vi "Main.vi"() -> ()   [LabVIEW 2019]
doc: "The myRIO Project template acquires acceleration data from the onboard accelerometer and displays the changes of acceleration values in a waveform chart."
uses:
  D:/PLIKI/INZYNIERKA/PROGRAM/STARE/EnumMS.ctl
panel:
  in  "ROZPOCZNIJ":bool caption="START"
  out "Error":bool
  in  "START":bool
  out "PRZEBIEG PREDKOŚCI OBROTOWEJ":dbl(graph)
  in  "Metody pomiarowe":T1(tab)
  in  "Rozdzielczość":dbl
  in  "Stała napieciowa":dbl
  out "Ścieżka zapisu danych":string
  out "Run":bool
  in  "ZATRZYMAJ":bool
  in  "STOP":bool
  out "Aktualna pedkosć obrotowa":dbl
  in  "Czas pomiaru":dbl
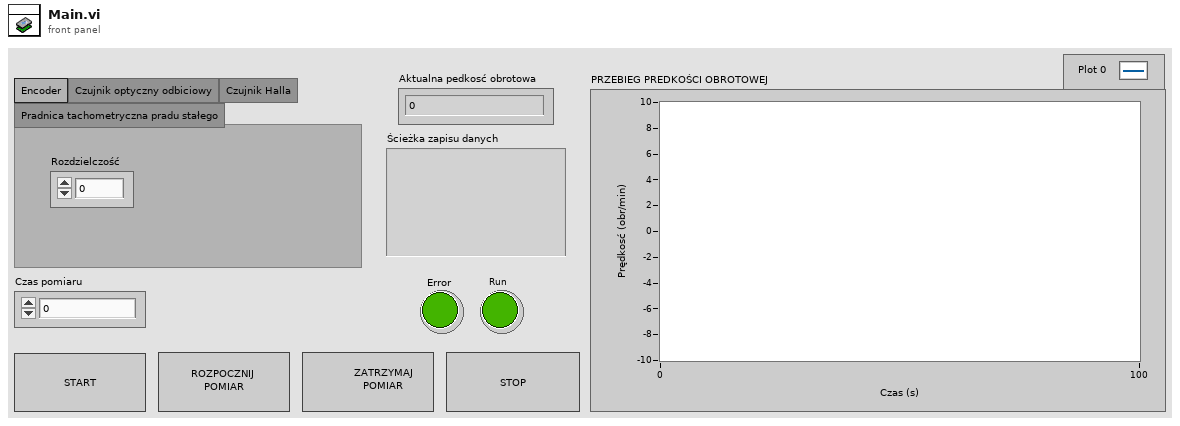
[diagram p1: front panel]
types:
  T1 = enum32{"Encoder", "Czujnik optyczny odbiciowy", "Czujnik Halla", "Pradnica tachometryczna pradu stałego"}
  T2 = enum16{"open", "open or create", "create or replace", "create", "open (read-only)"}
  T3 = cluster{"Rozczielczość enkoder":dbl, "Stał tachopradnicy":dbl, "RPM":dbl, "Nowa seria?":bool, "Error":bool, "Wybrana metoda":u8}
  T4 = typedef "EnumMS.ctl" = enum16{"Wait", "Method", "File", "Pouse/Start", "Aquisition", "Analysis", "Data", "Time Check"}
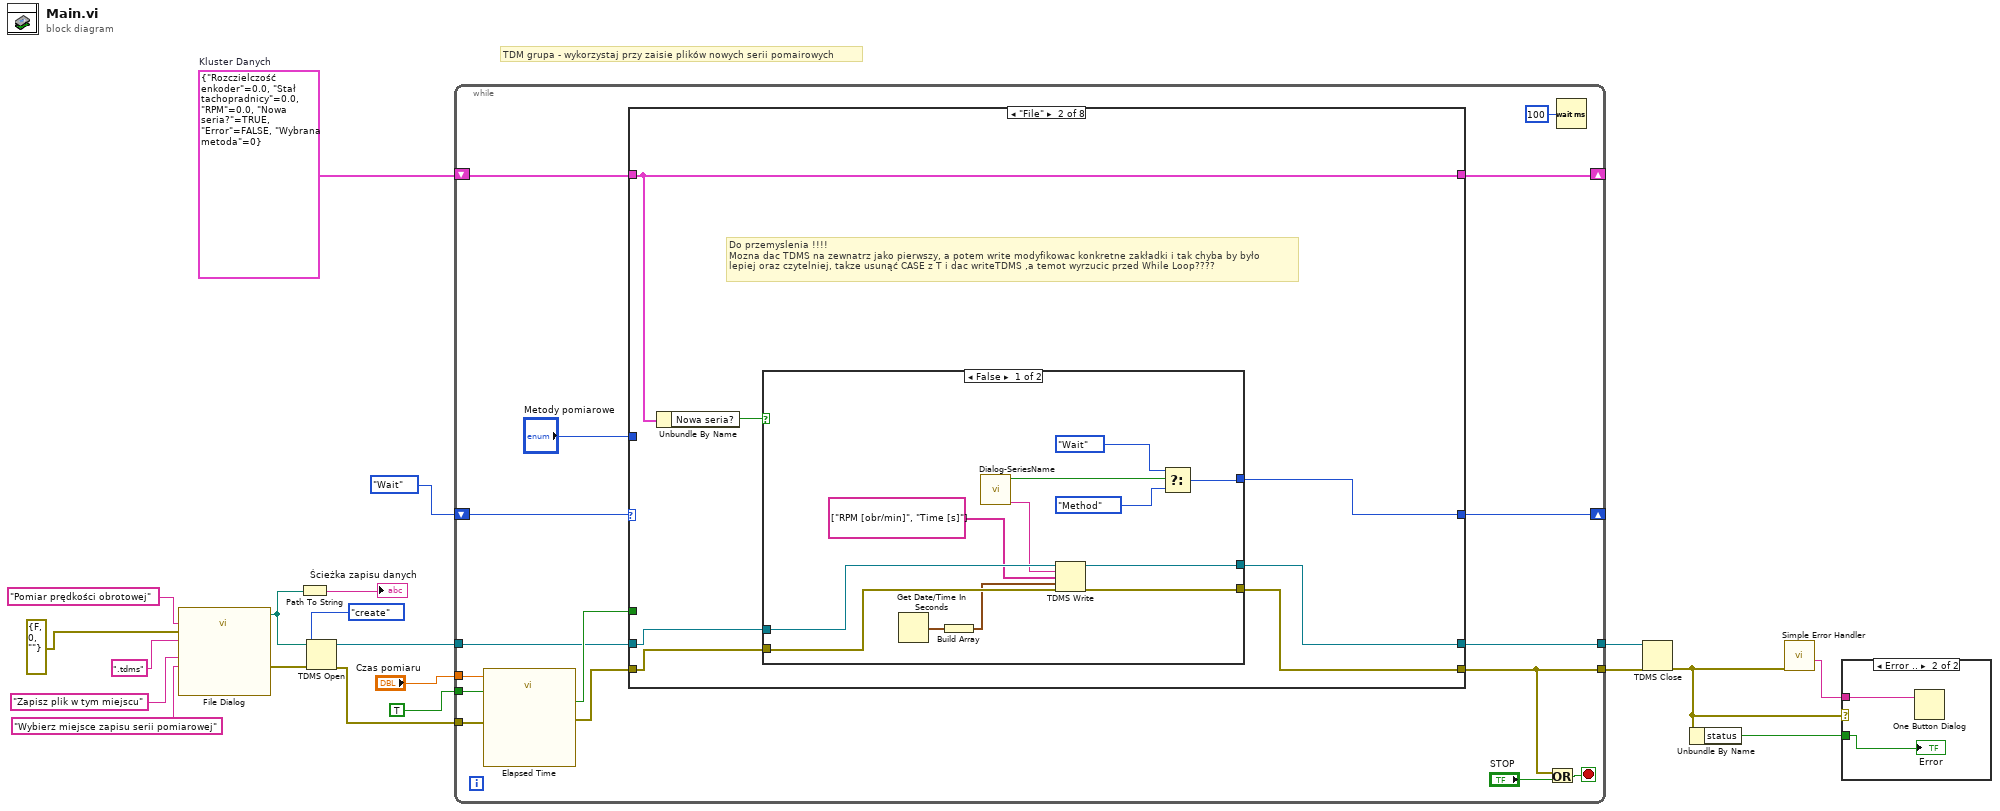
[diagram p0: block diagram]
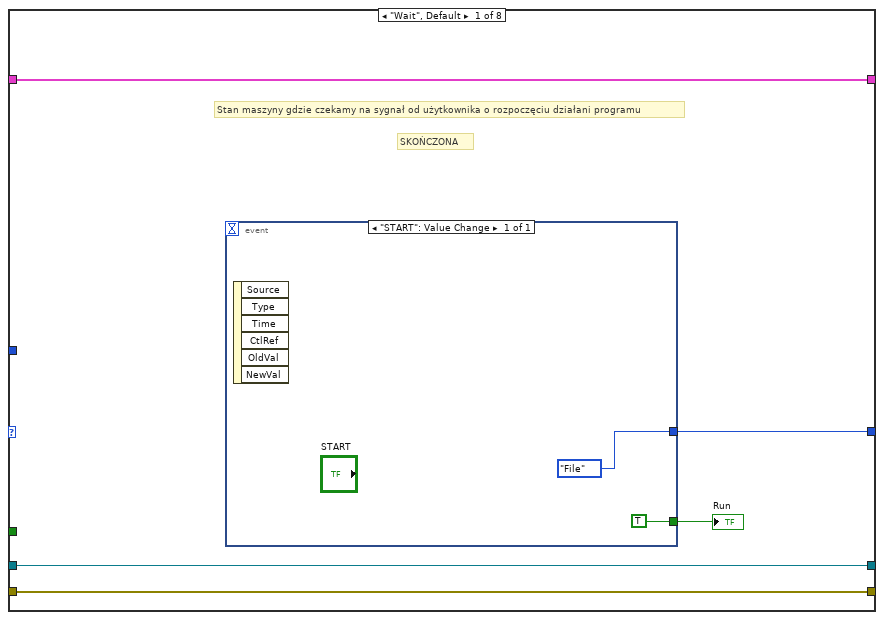
[diagram p3: hidden frame]
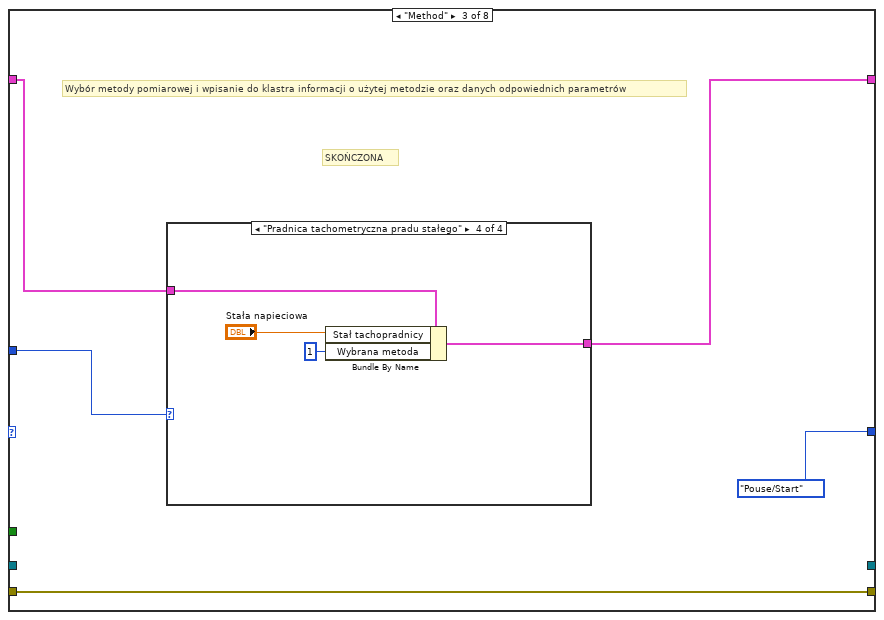
[diagram p5: hidden frame]
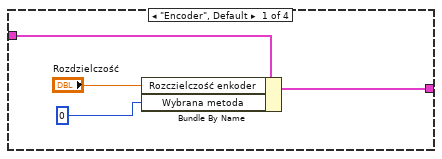
[diagram p6: hidden frame]
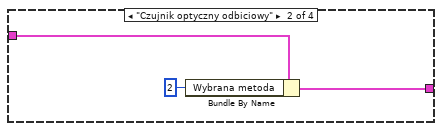
[diagram p7: hidden frame]
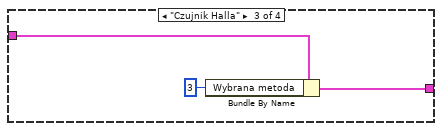
[diagram p8: hidden frame]
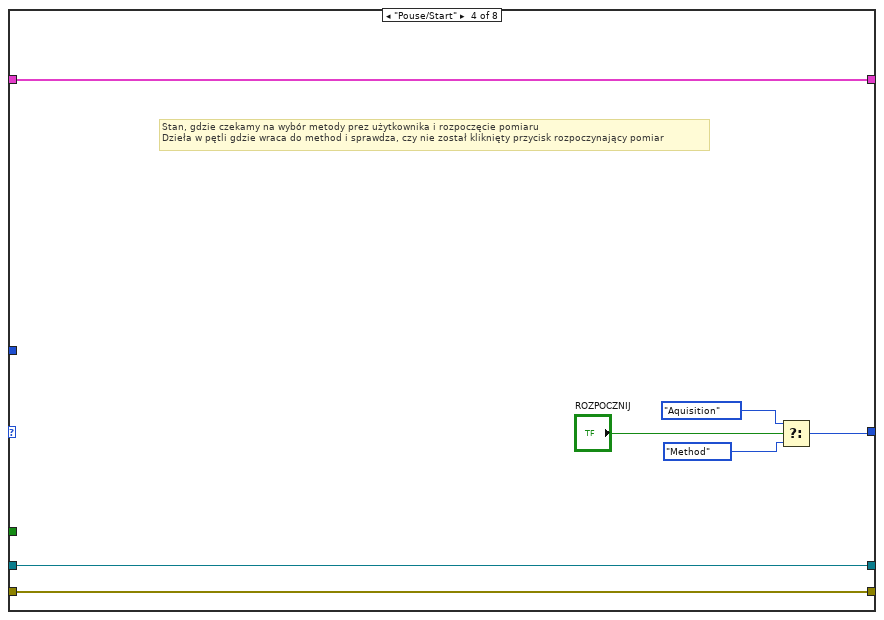
[diagram p9: hidden frame]
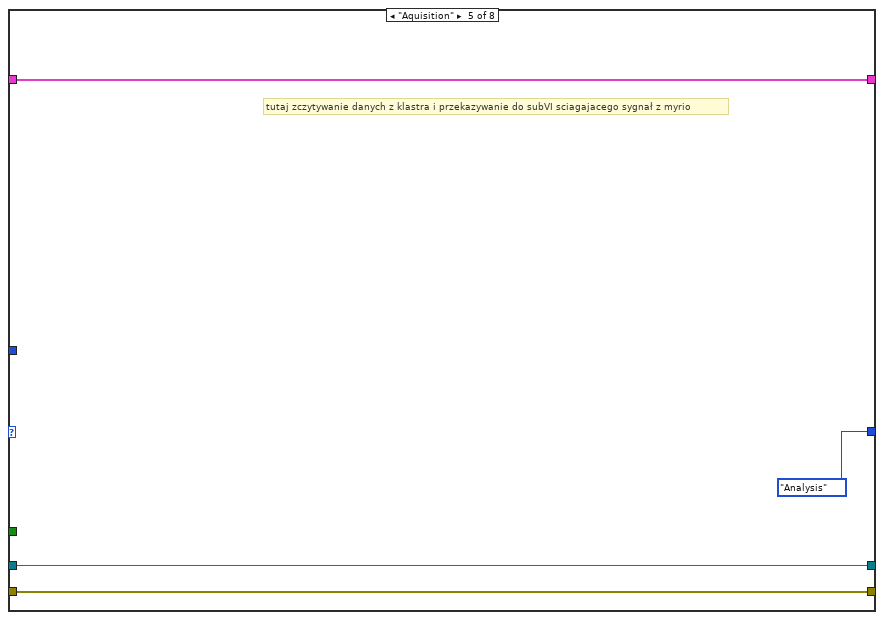
[diagram p10: hidden frame]
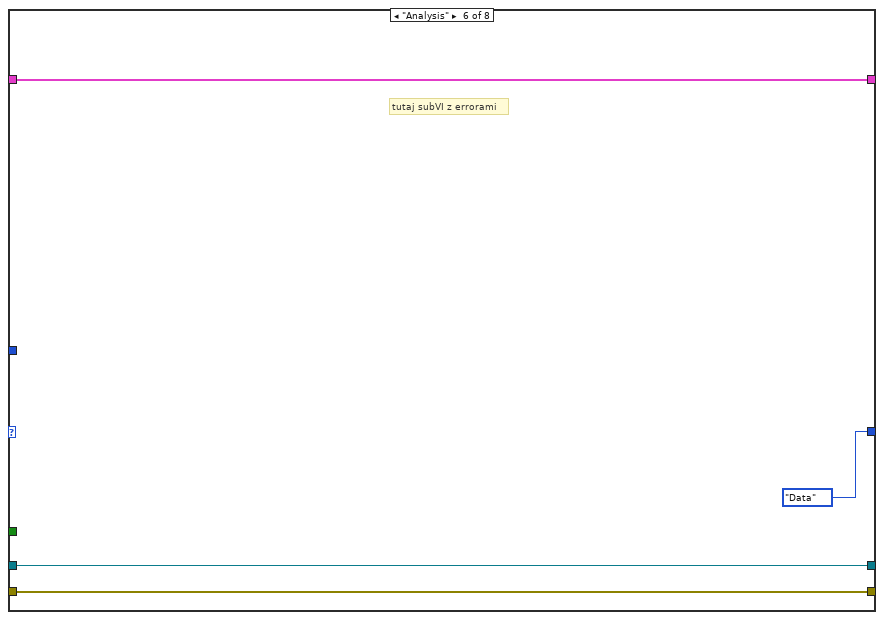
[diagram p11: hidden frame]
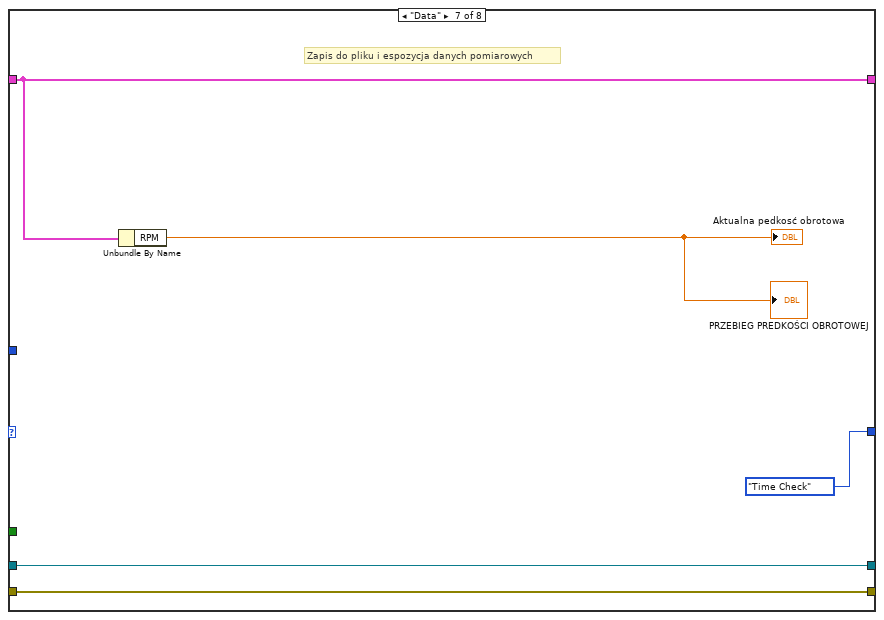
[diagram p12: hidden frame]
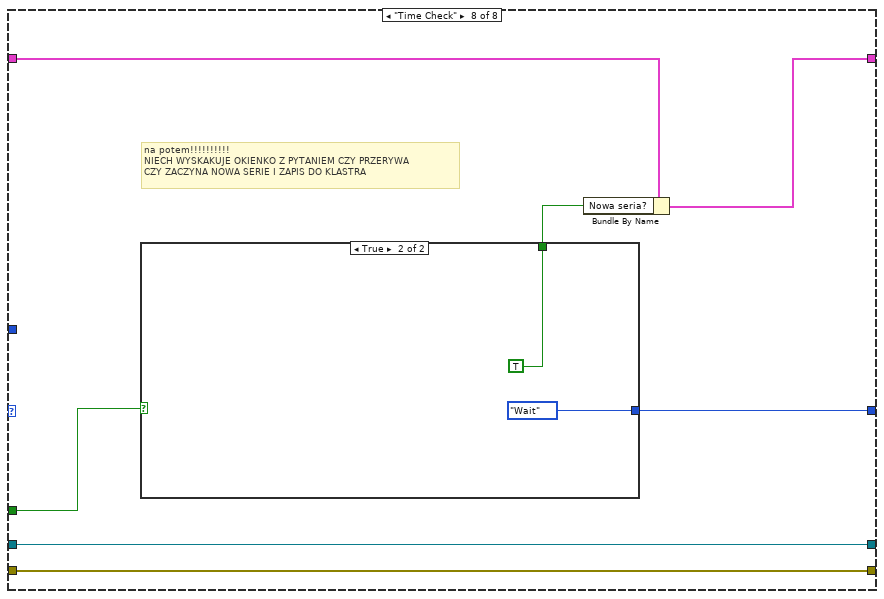
[diagram p13: hidden frame]
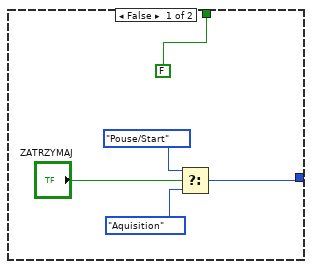
[diagram p14: hidden frame]
diagram:
  w13 = T3 {"Rozczielczość enkoder"=0.0, "Stał tachopradnicy"=0.0, "RPM"=0.0, "Nowa seria?"=TRUE, "Error"=FALSE, "Wybrana metoda"=0}  # Kluster Danych
  # "TDM grupa - wykorzystaj przy zaisie plików nowych serii pomairowych"
  n1 = call "File Dialog"("prompt"="Wybierz miejsce zapisu serii pomiarowej", "button label"="Zapisz plik w tym miejscu", "default name"="Pomiar prędkości obrotowej", "error in"=errorcluster {"status"=FALSE, "code"=0, "source"=""} ("error constant"), "pattern (all files)"=".tdms") -> ("selected path"=w6:path, "error out"=w4:errorcluster)  [unwired: 7 in, 2 out]
  n2 = Path To String(path=w6) -> (string=→"Ścieżka zapisu danych":string)
  n3 = TDMS Open(8:w4, 10:T2."create" ("operation (0:open)"), 11:w6) -> (0:w3:errorcluster, 3:w5:refnum<k34>)  [unwired: 4 in]
  n4 = while {
    shift-right: [w32] -> _
    shift-left: EnumMS."Wait" ("Stany") -> [w33]
    tunnel: "Czas pomiaru" -> [w31]
    tunnel: TRUE ("Reset") -> [w30]
    tunnel: [w26] -> w17
    shift-right: [w24] -> _
    shift-left: w13 -> [w25]
    tunnel: w5 -> [w22]
    tunnel: w3 -> [w23]
    tunnel: [w21] -> w1
    stop <- w34 stop-if-true
    n5 = call "Elapsed Time"("Time Target (s)"=w31, "Reset"=w30, "error in (no error)"=w23) -> ("Time has Elapsed"=w28:bool, "error out"=w27:errorcluster)  [unwired: 9 in, 6 out]
    n6 = case shown="\"File\"" w33 {
      tunnel: [w41 w44 EnumMS."Pouse/Start" ("Stany") w85 EnumMS."Analysis" ("Stany") EnumMS."Data" ("Stany") EnumMS."Time Check" ("Stany") w107] -> w32
      tunnel: "Metody pomiarowe" -> [_ _ w67 _ _ _ _ _]
      tunnel: w28 -> [_ _ _ _ _ _ _ w108]
      tunnel: w27 -> [w39 w48 w65 w84 w91 w96 w101 w106]
      tunnel: [w39 w46 w65 w84 w91 w96 w101 w106] -> w26
      tunnel: w25 -> [w38 w49 w64 w83 w90 w94 w99 w105]
      tunnel: [w38 w49 w63 w83 w90 w94 w99 w103] -> w24
      tunnel: w22 -> [w37 w47 _ w82 w89 w93 w97 w102]
      tunnel: [w37 w45 _ w82 w89 w93 w97 w102] -> w21
      frame "Wait", Default {
        # "SKOŃCZONA"
        # "Stan maszyny gdzie czekamy na sygnał od użytkownika o rozpoczęciu działani programu"
        n7 = event shown="[0] \"START\": Value Change" {
          selector: _ -> [_]
          dyn-events: _ -> [_]
          timeout: _ -> [_]
          tunnel: [EnumMS."File" ("Stany")] -> w41
          tunnel: [TRUE ("Run")] -> w40
          event "START": Value Change {
            n8 = event-data() -> ()  [unwired: 1 in, 6 out]
          }
        }
        "Run" <- w40
      }
      frame "File" {
        # "Do przemyslenia !!!!\nMozna dac TDMS na zewnatrz jako pierwszy, a potem write modyfikowac konkretne zakładki i tak chyba by było\nlepiej oraz czytelniej, takze usunąć CASE z T i dac writeTDMS ,a temot wyrzucic przed While Loop????"
        n9 = Unbundle By Name(w49) -> ("Nowa seria?"=w50:bool)
        n10 = case shown="False" w50 {
          tunnel: w48 -> [w61 _]
          tunnel: w47 -> [w60 _]
          tunnel: [w57 _] -> w46
          tunnel: [w56 _] -> w45
          tunnel: [w51 _] -> w44
          frame False {
            n11 = Get Date/Time In Seconds() -> (seconds since 1Jan1904=w62:timestamp)
            n12 = Build Array(w62) -> (w59:timestamp[])
            n13 = call "Dialog-SeriesName.vi"() -> ("String"=w55:string, "Anulowane?"=w54:bool)  [unwired: 10 in]
            n14 = TDMS Write(0:w60, 5:w55, 7:string[] ["RPM [obr/min]", "Time [s]"] ("channel name(s) in (Untitled)"), 9:w59, 11:w61) -> (4:w56:refnum<k34>, 15:w57:errorcluster)  [unwired: 1 in, 2 out]
            n15 = Select(t=EnumMS."Wait" ("Stany"), s=w54, f=EnumMS."Method" ("Stany")) -> (s? t:f=w51:T4)
          }
          frame True {
          }
        }
      }
      frame "Method" {
        # "SKOŃCZONA"
        # "Wybór metody pomiarowej i wpisanie do klastra informacji o użytej metodzie oraz danych odpowiednich parametrów"
        n16 = case shown="\"Pradnica tachometryczna pradu stałego\"" w67 {
          tunnel: w64 -> [w70 w74 w77 w81]
          tunnel: [w71 w73 w76 w79] -> w63
          frame "Encoder", Default {
            n17 = Bundle By Name(cluster=w70, "Rozczielczość enkoder"="Rozdzielczość", "Wybrana metoda"=u8 0) -> (w71:T3)
          }
          frame "Czujnik optyczny odbiciowy" {
            n18 = Bundle By Name(cluster=w74, "Wybrana metoda"=u8 2) -> (w73:T3)
          }
          frame "Czujnik Halla" {
            n19 = Bundle By Name(cluster=w77, "Wybrana metoda"=u8 3) -> (w76:T3)
          }
          frame "Pradnica tachometryczna pradu stałego" {
            n20 = Bundle By Name(cluster=w81, "Stał tachopradnicy"="Stała napieciowa", "Wybrana metoda"=u8 1) -> (w79:T3)
          }
        }
      }
      frame "Pouse/Start" {
        # "Stan, gdzie czekamy na wybór metody prez użytkownika i rozpoczęcie pomiaru\nDzieła w pętli gdzie wraca do method i sprawdza, czy nie został kliknięty przycisk rozpoczynający pomiar"
        n21 = Select(t=EnumMS."Aquisition" ("Stany"), s="ROZPOCZNIJ", f=EnumMS."Method" ("Stany")) -> (s? t:f=w85:T4)
      }
      frame "Aquisition" {
        # "tutaj zczytywanie danych z klastra i przekazywanie do subVI sciagajacego sygnał z myrio"
      }
      frame "Analysis" {
        # "tutaj subVI z errorami"
      }
      frame "Data" {
        # "Zapis do pliku i espozycja danych pomiarowych"
        n22 = Unbundle By Name(w99) -> ("RPM"=→"PRZEBIEG PREDKOŚCI OBROTOWEJ" →"Aktualna pedkosć obrotowa":dbl)
      }
      frame "Time Check" {
        # "na potem!!!!!!!!!!\nNIECH WYSKAKUJE OKIENKO Z PYTANIEM CZY PRZERYWA\nCZY ZACZYNA NOWA SERIE I ZAPIS DO KLASTRA"
        n23 = case shown="True" w108 {
          tunnel: [w111 EnumMS."Wait" ("Stany")] -> w107
          tunnel: [FALSE TRUE] -> w104
          frame False {
            n24 = Select(t=EnumMS."Pouse/Start" ("Stany"), s="ZATRZYMAJ", f=EnumMS."Aquisition" ("Stany")) -> (s? t:f=w111:T4)
          }
          frame True {
          }
        }
        n25 = Bundle By Name(cluster=w105, "Nowa seria?"=w104) -> (w103:T3)
      }
    }
    n26 = Or(x=w26, y="STOP") -> (x .or. y?=w34:bool)
    n27 = Wait (ms)(milliseconds to wait=u32 100) -> ()  [unwired: 1 out]
  }
  n28 = TDMS Close(8:w17, 11:w1) -> (0:w14:errorcluster)  [unwired: 1 out]
  n29 = Unbundle By Name(w14) -> ("status"=w15:bool)
  n30 = call <vilib>:"Simple Error Handler.vi"("error in (no error)"=w14) -> ("source out"=w16:string)  [unwired: 4 in, 4 out]
  n31 = case shown="Error .." w14 {
    tunnel: w16 -> [_ w117]
    tunnel: w15 -> [_ w116]
    frame No Error {
    }
    frame Error {
      n32 = One Button Dialog(message=w117) -> ()  [unwired: 1 in, 1 out]
      "Error" <- w116
    }
  }
